vi "AssetMgrGetMissingChannelsFromHardwareRequest_Create.vi"(7 "Header":T15, 8 "error in (no error)":errorcluster, 9 "AssetMgrGetMissingChannelsFromHardwareRequest":T1, 11 "ReplyTo":string) -> (0 "error out":errorcluster, 3 "Message":T16)   [LabVIEW 2017]
uses:
  <vilib>/addons/InsightCM/MessageBus/Base/controls/Message.ctl
  <vilib>/addons/InsightCM/MessageBus/Base/controls/MessageHeader.ctl
  <vilib>/addons/InsightCM/MessageBus/Base/controls/KeyValuePair.ctl
  <vilib>/addons/InsightCM/MessageBus/MessageLibrary/AssetManager/controls/AssetMgrGetMissingChannelsFromHardwareRequestBody.ctl
  <vilib>/addons/InsightCM/MessageBus/Base/controls/DeviceModel.ctl
  <vilib>/addons/InsightCM/MessageBus/Base/controls/Device.ctl
  <vilib>/addons/InsightCM/MessageBus/Base/controls/DeviceState.ctl
  <vilib>/addons/InsightCM/MessageBus/Base/controls/DataGroup.ctl
  <vilib>/addons/InsightCM/MessageBus/Base/controls/BurstModeTrigger.ctl
  <vilib>/addons/InsightCM/MessageBus/Base/controls/Trigger.ctl
  <vilib>/addons/InsightCM/MessageBus/Base/controls/Condition.ctl
  <vilib>/addons/InsightCM/MessageBus/Base/controls/DeviceSensorGroup.ctl
  <vilib>/addons/InsightCM/MessageBus/Base/controls/WirelessEndpoint.ctl
  <vilib>/addons/InsightCM/MessageBus/Base/controls/WirelessChannel.ctl
  <vilib>/addons/InsightCM/MessageBus/Base/controls/Channel.ctl
  <vilib>/addons/InsightCM/MessageBus/Base/controls/Tag.ctl
  <vilib>/addons/InsightCM/MessageBus/Base/controls/MessageClassType.ctl
  <vilib>/addons/InsightCM/Utilities/PropertyHelpers/PropertyHelpers.lvlib
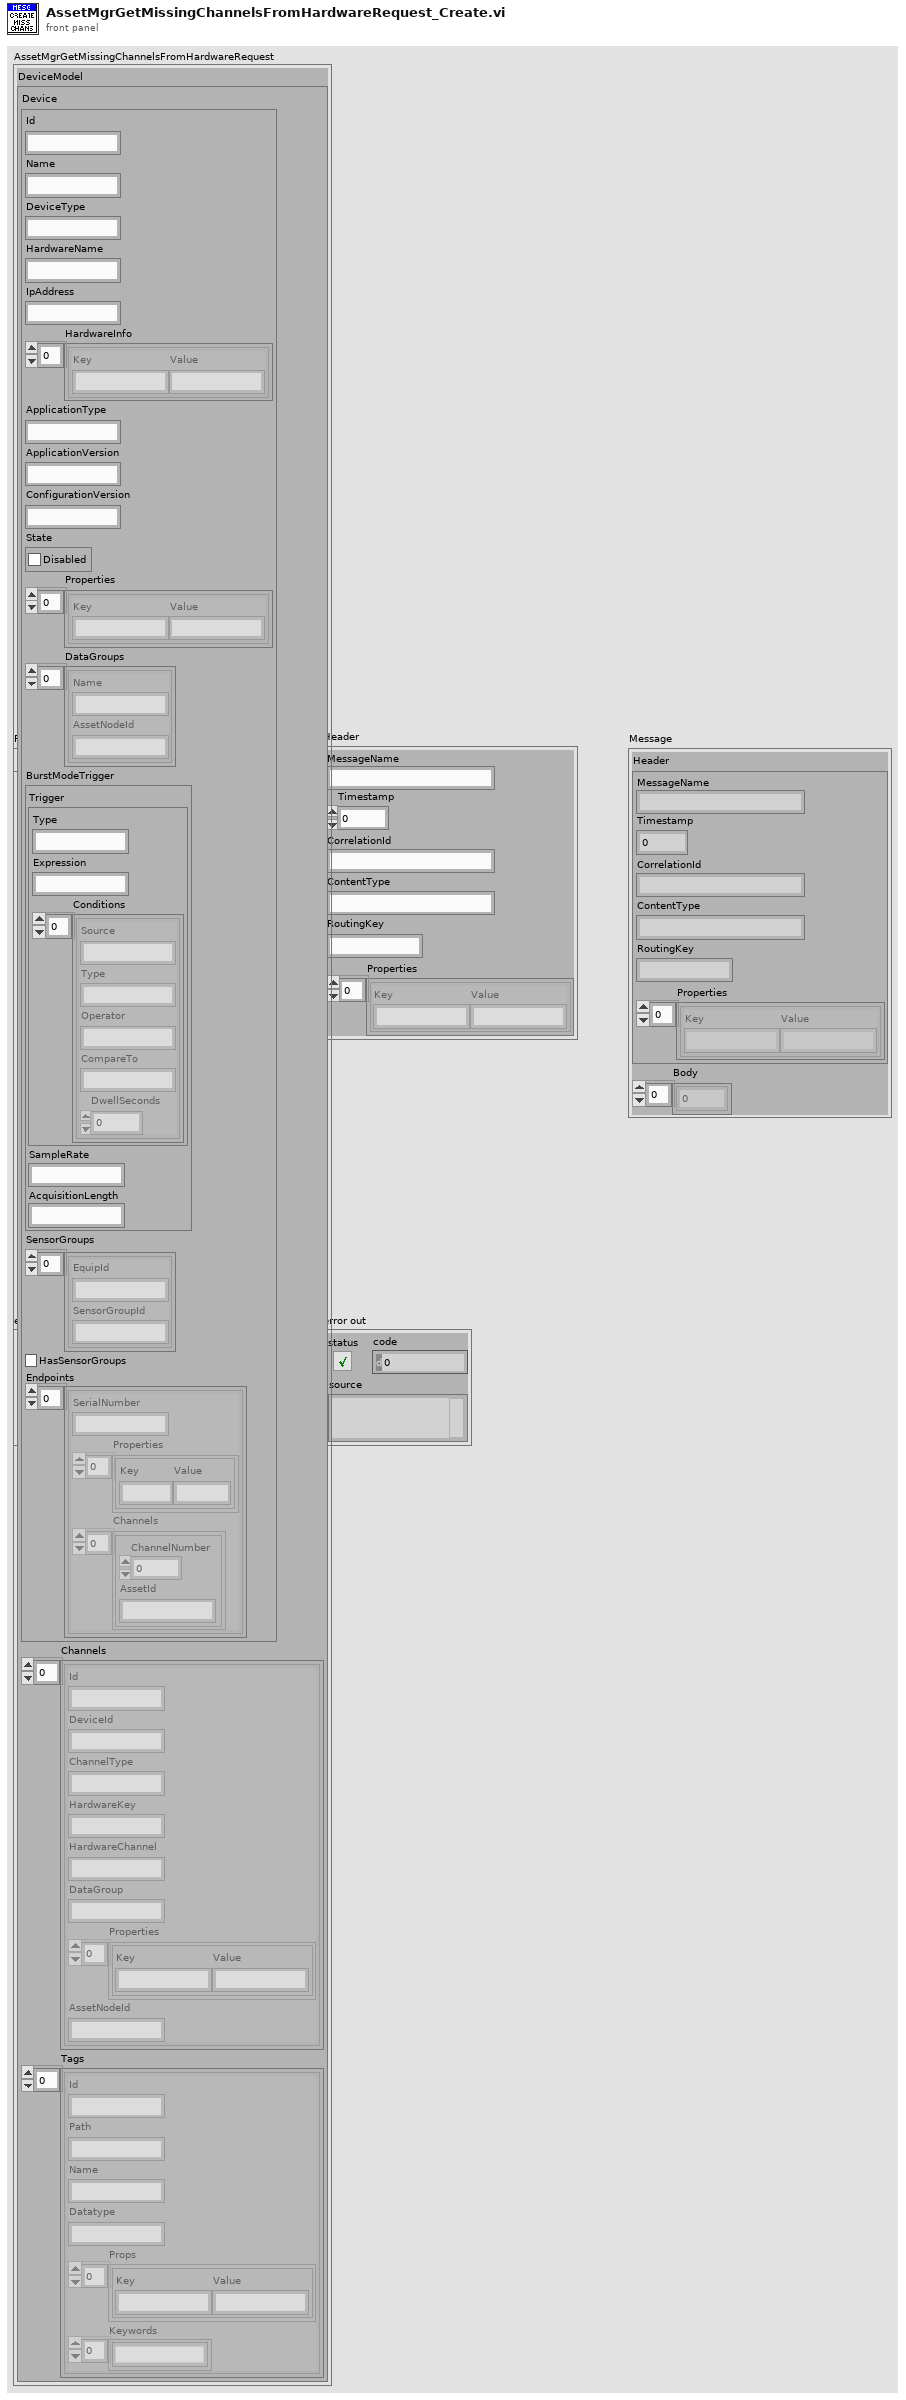
[diagram p1: front panel]
types:
  T1 = typedef "AssetMgrGetMissingChannelsFromHardwareRequestBody.ctl" = cluster{"DeviceModel":T2}
  T2 = typedef "DeviceModel.ctl" = cluster{"Device":T3, "Channels":T13[], "Tags":T14[]}
  T3 = typedef "Device.ctl" = cluster{"Id":string, "Name":string, "DeviceType":string, "HardwareName":string, "IpAddress":string, "HardwareInfo":T4[], "ApplicationType":string, "ApplicationVersion":string, "ConfigurationVersion":string, "State":T5, "Properties":T4[], "DataGroups":T6[], "BurstModeTrigger":T7, "SensorGroups":T10[], "HasSensorGroups":bool, "Endpoints":T11[]}
  T4 = typedef "KeyValuePair.ctl" = cluster{"Key":string, "Value":string}
  T5 = typedef "DeviceState.ctl" = cluster{"Disabled":bool}
  T6 = typedef "DataGroup.ctl" = cluster{"Name":string, "AssetNodeId":string}
  T7 = typedef "BurstModeTrigger.ctl" = cluster{"Trigger":T8, "SampleRate":string, "AcquisitionLength":string}
  T8 = typedef "Trigger.ctl" = cluster{"Type":string, "Expression":string, "Conditions":T9[]}
  T9 = typedef "Condition.ctl" = cluster{"Source":string, "Type":string, "Operator":string, "CompareTo":string, "DwellSeconds":dbl}
  T10 = typedef "DeviceSensorGroup.ctl" = cluster{"EquipId":string, "SensorGroupId":string}
  T11 = typedef "WirelessEndpoint.ctl" = cluster{"SerialNumber":string, "Properties":T4[], "Channels":T12[]}
  T12 = typedef "WirelessChannel.ctl" = cluster{"ChannelNumber":i32, "AssetId":string}
  T13 = typedef "Channel.ctl" = cluster{"Id":string, "DeviceId":string, "ChannelType":string, "HardwareKey":string, "HardwareChannel":string, "DataGroup":string, "Properties":T4[], "AssetNodeId":string}
  T14 = typedef "Tag.ctl" = cluster{"Id":string, "Path":string, "Name":string, "Datatype":string, "Props":T4[], "Keywords":string[]}
  T15 = typedef "MessageHeader.ctl" = cluster{"MessageName":string, "Timestamp":i64, "CorrelationId":string, "ContentType":string, "RoutingKey":string, "Properties":T4[]}
  T16 = typedef "Message.ctl" = cluster{"Header":T15, "Body":u8[]}
  T17 = typedef "MessageClassType.ctl" = enum16{"Request", "Response", "Broadcast", "RoutedMessage"}
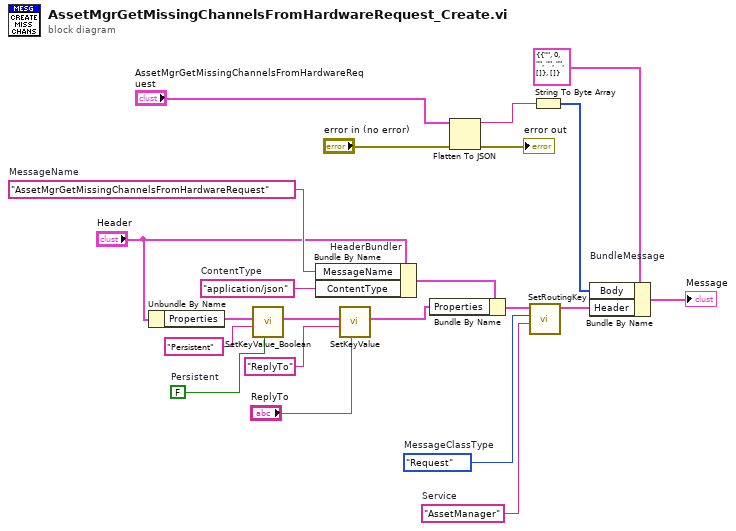
[diagram p0: block diagram]
diagram:
  w18 = MessageClassType."Request"  # MessageClassType
  w3 = "AssetManager"  # Service
  w13 = FALSE  # Persistent
  w19 = "AssetMgrGetMissingChannelsFromHardwareRequest"  # MessageName
  w16 = "application/json"  # ContentType
  n1 = Unbundle By Name("Header") -> ("Properties"=w15:T4[])
  n2 = call <vilib>:"SetKeyValue_Boolean.vi"("value"=w13, "key"="Persistent" ("Key"), "key value pairs"=w15) -> ("key value pairs out"=w11:T4[])  [unwired: 8 in]
  n3 = Bundle By Name "HeaderBundler"(cluster="Header", "MessageName"=w19, "ContentType"=w16) -> (w9:T15)
  n4 = call <vilib>:"SetKeyValue.vi"("value"="ReplyTo", "key"="ReplyTo" ("Key"), "key value pairs"=w11) -> ("key value pairs out"=w8:T4[])  [unwired: 8 in]
  n5 = Bundle By Name(cluster=w9, "Properties"=w8) -> (w10:T15)
  n6 = Flatten To JSON(anything="AssetMgrGetMissingChannelsFromHardwareRequest", error in (no error)="error in (no error)") -> (JSON string=w2:string, 11:→"error out":errorcluster)  [unwired: 1 in]
  n7 = call <vilib>:"SetRoutingKey.vi"("SendTo"=w3, "MessageClassType"=w18, "Message Header in"=w10) -> ("Message Header out"=w12:T15)  [unwired: 8 in]
  n8 = String To Byte Array(string=w2) -> (unsigned byte array=w21:u8[])
  n9 = Bundle By Name "BundleMessage"(cluster=T16 {"Header"={"MessageName"="", "Timestamp"=0, "CorrelationId"="", "ContentType"="", "RoutingKey"="", "Properties"=[]}, "Body"=[]} ("Message"), "Body"=w21, "Header"=w12) -> (→"Message":T16)
